vi "Element Events.vi"(8 "error in (no error)":errorcluster, 11 "HtmlButtonControl in":refnum<class "HttpButtonControl.lvclass">) -> (0 "error out":errorcluster, 2 "Element Events":refnum<class "Control Event Registrations.lvclass">, 3 "HtmlButtonControl out":refnum<class "HttpButtonControl.lvclass">)   [LabVIEW 2020, in "VolatusGUIElements.lvlib" / "HttpButtonControl.lvclass"]
uses:
  HttpButtonControl.lvclass
  C:/dev/lv20CE/relink/lv-volatus/VolatusGUI/OnValueChangeHandler/OnValueChangeHandler.lvclass
  VolatusGUI/Control Event Registrations/Control Event Registrations.lvclass
  HttpButtonControl.lvclass/HttpButtonControl.ctl
  C:/dev/lv20CE/relink/lv-volatus/VolatusGUI/GUI Element/GUI Element.lvclass
  C:/dev/lv20CE/relink/lv-volatus/VolatusGUIElements/HttpButtonControl/HttpButtonControl.lvclass
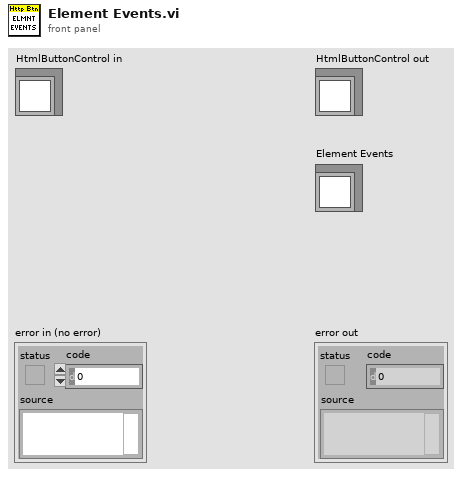
[diagram p1: front panel]
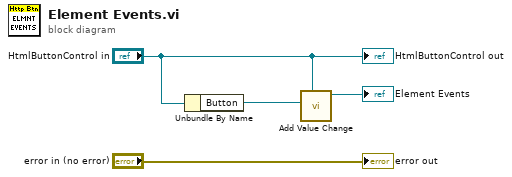
[diagram p0: block diagram]
diagram:
  n1 = Unbundle By Name("HtmlButtonControl in") -> ("Button"=w1:refnum<vi>)
  n2 = call "Add Value Change.vi"("Control"="HtmlButtonControl in", "CtlRef"=w1) -> ("Control Event Registrations out"=→"Element Events":refnum<class "Control Event Registrations.lvclass">)  [unwired: 8 in, 1 out]
  "error out" <- "error in (no error)"
  "HtmlButtonControl out" <- "HtmlButtonControl in"
